vi "StopAllProcesses.vi"(8 "error in (no error)":errorcluster) -> (0 "error out":errorcluster)   [LabVIEW 2013]
uses:
  030 - EVENTS/EnumFgvEventCommand.ctl
  030 - EVENTS/04 - ToAllProcesses/ToAllProcessesEvent.ctl
  030 - EVENTS/04 - ToAllProcesses/EnumToAllProcessesCommand.ctl
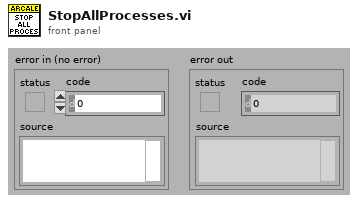
[diagram p1: front panel]
types:
  T1 = typedef "EnumToAllProcessesCommand.ctl" = enum16{"Stop all processes", "Autotest"}
  T2 = typedef "ToAllProcessesEvent.ctl" = cluster{"Command":T1}
  T3 = typedef "EnumFgvEventCommand.ctl" = enum16{"Setup", "Cleanup", "Get"}
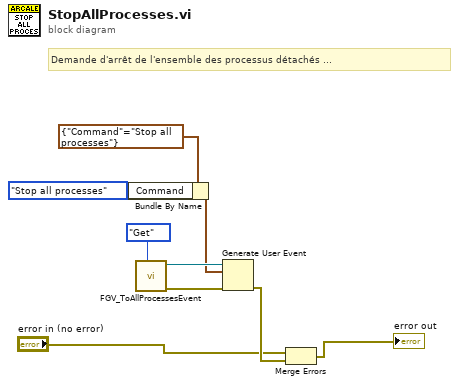
[diagram p0: block diagram]
diagram:
  # "Demande d'arrêt de l'ensemble des processus détachés ..."
  n1 = Bundle By Name(cluster=T2 {"Command"=enum."Stop all processes"} ("event data"), "Command"=EnumToAllProcessesCommand."Stop all processes") -> (w5:T2)
  n2 = call "FGV_ToAllProcessesEvent.vi"("Command"=EnumFgvEventCommand."Get") -> ("error out"=w8:errorcluster, "ToAllProcessesEvent"=w7:refnum<user-event>)  [unwired: 9 in]
  n3 = Generate User Event(user event=w7, event data cluster=w5, error in=w8) -> (error out=w3:errorcluster)  [unwired: 1 in, 1 out]
  n4 = Merge Errors("error in (no error)", w3) -> (→"error out":errorcluster)
